vi "enumerateStaticDependencies.vi"(8 "error in (no error)":errorcluster, 11 "SMO.UI.Example":refnum<class "SMO.UI.Example.lvclass">) -> (0 "error out":errorcluster, 2 "Static Dependencies":refnum<class "Dependency.lvclass">[](array[class]), 3 "SMO.UI.Example out":refnum<class "SMO.UI.Example.lvclass">)   [LabVIEW 2013, in "SMO.UI.Example.lvclass"]
uses:
  SMO.UI.Example.lvclass
  Dependency/Dependency.lvclass
  Typedefs/Dependencies--Cluster.ctl
  SMO.Example/SMO.Example.lvclass
  SMO.UI/SMO.UI.lvclass
  SMO/SMO.lvclass
panel:
  # "For instructions on how to use the JKI State Machine Objects, examples and video tutorials, visit:\nhttp://jki.net/state-machine-objects/\n\nJKI State Machine Objects™\nhttp://jki.net/state-machine-objects/\nCopyright (C) 2005-2015, JKI <info@jki.net>\nALL RIGHTS RESERVED"
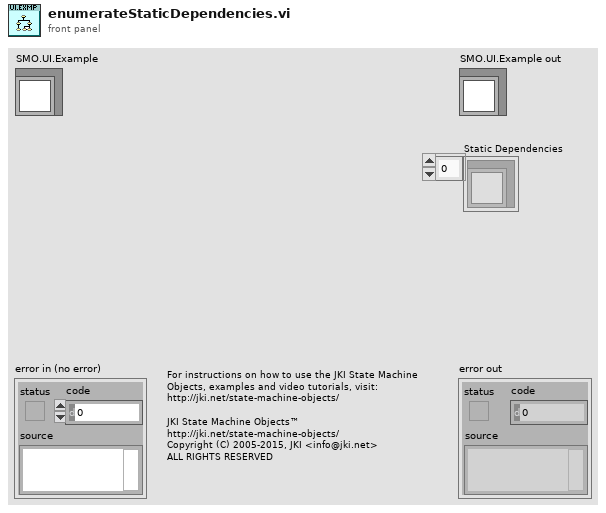
[diagram p1: front panel]
types:
  T1 = typedef "SMO.UI.Example.lvclass/Dependencies--Cluster.ctl" = cluster{"SMO.Example":refnum<class "SMO.Example.lvclass">}
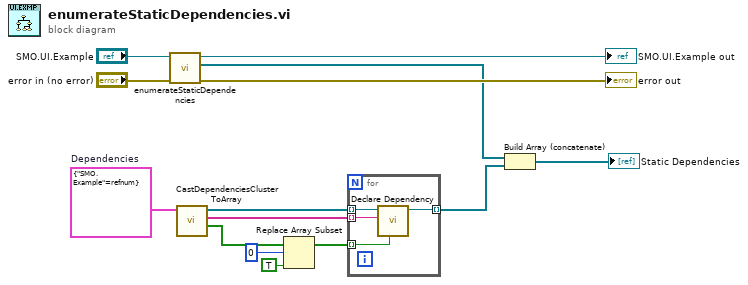
[diagram p0: block diagram]
diagram:
  w3 = T1 {"SMO.Example"=refnum}  # Dependencies
  n1 = call-parent "enumerateStaticDependencies.vi"("error in (no error)"="error in (no error)", "SMO"="SMO.UI.Example") -> ("error out"=→"error out":errorcluster, "Static Dependencies"=w2:refnum<class "Dependency.lvclass">[], "SMO out"=→"SMO.UI.Example out":refnum<class "SMO.UI.Example.lvclass">)  [unwired: 7 in]
  n2 = call "CastDependenciesClusterToArray.vi"("Dependencies Cluster"=w3) -> ("Shared Resources"=w5:bool[], "Dependencies Names"=w9:string[], "Dependencies Array"=w10:refnum<class "SMO.lvclass">[])  [unwired: 8 in]
  n3 = Replace Array Subset(array=w5, new element=TRUE ("Shared Resource (F)"), index=0) -> (w4:bool[])
  n4 = for {
    tunnel: [w18] -> w8 mode=indexing
    tunnel: w10 -> [w17] mode=indexing
    tunnel: w9 -> [w16] mode=indexing
    tunnel: w4 -> [w15] mode=indexing
    n5 = call "Declare Dependency.vi"("Shared Resource (F)"=w15, "Name"=w16, "Type"=w17) -> ("Dependency out"=w18:refnum<class "Dependency.lvclass">)  [unwired: 7 in, 1 out]
  }
  n6 = Build Array (concatenate)(w2, w8) -> (→"Static Dependencies":refnum<class "Dependency.lvclass">[])
